vi "Runtime beenden.vi"(9 "Zustand":T1=enum."Exit") -> (1 "Zustand":T1)   [LabVIEW 2020, in "allgemeine Sub-VIs.lvlib"]
uses:
  allgemeine Sub-VIs.lvlib
  Visualisierungs Elemente/Button.ctl
  Funktionstasten/Zustaende.ctl
  Funktionstasten/Funktionstasten.lvlib
  Seiten/CalGas Aufschaltung/CalGas Aufschaltung.lvlib
panel:
  in  "Abbrechen":T2
  in  "Beenden":T2
  # "IAG Runtime herunterfahren!"
  # "Wie möchten Sie vorgehen?"
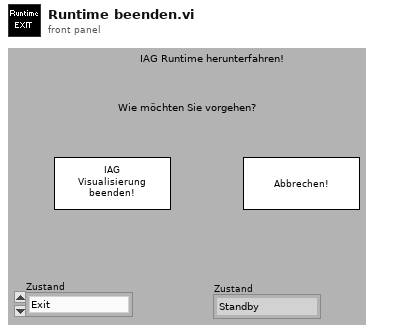
[diagram p1: front panel]
types:
  T1 = typedef "Funktionstasten.lvlib/Zustaende.ctl" = enum16{"Standby", "Pause", "Eco", "Messen", "Kalibrieren", "Spülen Filter", "Spülen Leitung", "Umgebungsluft", "0-Gas", "Cal-Gas", "CG zu PNS", "-------------", "Init 1", "Init 2", "Init 3", "Init 4", "Messen vorbereiten", "Messen durchführen", "Exit"}
  T2 = typedef "Button.ctl" = bool
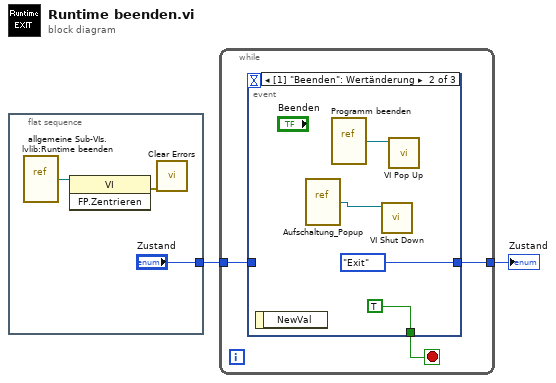
[diagram p0: block diagram]
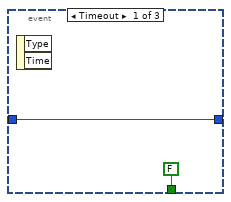
[diagram p2: hidden frame]
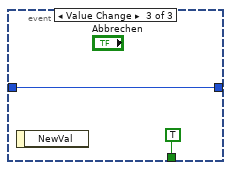
[diagram p3: hidden frame]
diagram:
  n1 = flat-sequence {
    tunnel: ["Zustand"] -> w2
    frame #0 {
      n2 = vi-ref "allgemeine Sub-VIs.lvlib:Runtime beenden.vi"() -> (w3:refnum<vi>)
      n3 = invoke class="VI" method="FP.Zentrieren"(reference=w3) -> (error out=w4:errorcluster)  [unwired: 2 in, 2 out]
      n4 = call <vilib>:"Clear Errors.vi"("error in (no error)"=w4) -> ()  [unwired: 5 in, 2 out]
    }
  }
  n5 = while {
    tunnel: w2 -> [w7]
    tunnel: [w6] -> w1
    stop <- w8 stop-if-true
    n6 = event shown="[1] \"Beenden\": Wertänderung" {
      selector: _ -> [_ _ _]
      dyn-events: _ -> [_ _ _]
      timeout: _ -> [_ _ _]
      tunnel: [FALSE TRUE TRUE] -> w8
      tunnel: w7 -> [w9 _ w15]
      tunnel: [w9 Zustaende."Exit" ("Zustand") w15] -> w6
      event Timeout {
        n7 = event-data() -> ()  [unwired: 1 in, 2 out]
      }
      event Value Change {
        n8 = event-data() -> ()  [unwired: 1 in, 1 out]
        n9 = vi-ref "Aufschaltung_Popup.vi"() -> (w11:refnum<vi>)
        n10 = vi-ref "Programm beenden.vi"() -> (w12:refnum<vi>)
        n11 = call "VI Shut Down.vi"("VI Referenz"=w11) -> ()  [unwired: 11 in]
        n12 = call "VI Pop Up.vi"("VI Referenz"=w12) -> ()  [unwired: 10 in, 1 out]
      }
      event Value Change {
        n13 = event-data() -> ()  [unwired: 1 in, 1 out]
      }
    }
  }
  "Zustand" <- w1
